vi "Timeout.vi"(1 "Timeout":u32, 2 "Initialize":bool) -> (0 "Timed Out?":bool)   [LabVIEW 2019]
uses:
  Command_Execution_State.ctl
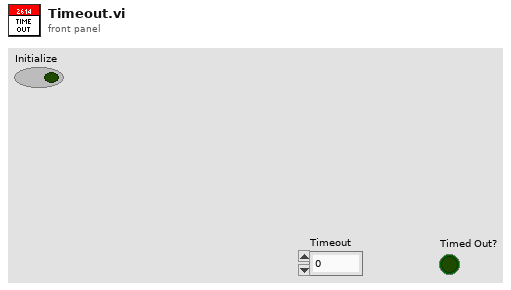
[diagram p1: front panel]
types:
  T1 = typedef "Command_Execution_State.ctl" = enum16{"Initialize", "Execute", "Finish"}
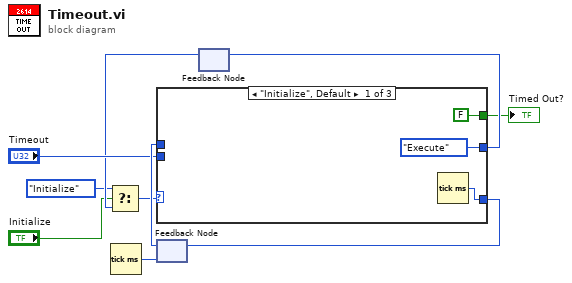
[diagram p0: block diagram]
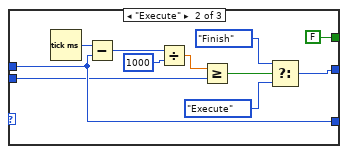
[diagram p2: hidden frame]
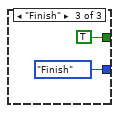
[diagram p3: hidden frame]
diagram:
  n1 = Tick Count (ms)() -> (millisecond timer value=w6:u32)
  n2 = feedback #1(w6) -> (w8:u32)
  n3 = feedback #2() -> (w4:T1)  [unwired: 1 in]
  n4 = Select(t=Command_Execution_State."Initialize", s="Initialize", f=w4) -> (s? t:f=w3:T1)
  n5 = case shown="\"Initialize\", Default" w3 {
    tunnel: [Command_Execution_State."Execute" w24 Command_Execution_State."Finish" ("t")] -> w10
    tunnel: [w13 w20 _] -> w9
    tunnel: w8 -> [_ w20 _]
    tunnel: "Timeout" -> [_ w18 _]
    tunnel: [FALSE FALSE TRUE] -> w5
    frame "Initialize", Default {
      n6 = Tick Count (ms)() -> (millisecond timer value=w13:u32)
    }
    frame "Execute" {
      n7 = Tick Count (ms)() -> (millisecond timer value=w21:u32)
      n8 = Subtract(x=w21, y=w20) -> (x-y=w17:u32)
      n9 = Divide(x=w17, y=u32 1000) -> (x/y=w15:dbl)
      n10 = Greater Or Equal?(x=w15, y=w18) -> (x >= y?=w19:bool)
      n11 = Select(t=Command_Execution_State."Finish", s=w19, f=Command_Execution_State."Execute" ("t")) -> (s? t:f=w24:T1)
    }
    frame "Finish" {
    }
  }
  "Timed Out?" <- w5
  n12 = feedback-in #1(w9) -> ()
  n13 = feedback-in #2(w10) -> ()
